vi "sub_main_mapgraph.vi"() -> (3 "graph ui array":T1(array[cluster]))   [LabVIEW 2019]
uses:
  Ctrl/waypoint_buf.ctl
  Ctrl/points.ctl
  Ctrl/pid-in-params.ctl
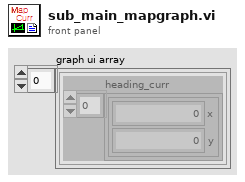
[diagram p1: front panel]
types:
  T1 = cluster{"heading_curr ":cluster{"x":dbl, "y":dbl}[]}[]
  T2 = cluster{"heading_curr ":cluster{"x":dbl, "y":dbl}[]}
  T3 = typedef "pid-in-params.ctl" = enum16{"read", "write"}
  T4 = typedef "points.ctl" = enum16{"read", "lookahead circle in", "lookahead in", "looktail in", "center in", "closest"}
  T5 = typedef "waypoint_buf.ctl" = enum16{"clear", "write", "read"}
  T6 = cluster{"deg_agv-lookahead":dbl, "deg_waypoint":dbl, "deg_gap":dbl, "deg_target":dbl, "pid output":dbl, "dis-gap":dbl, "deg_agv-center":dbl}
  T7 = cluster{"stop pt update out":cluster{dbl, dbl}[]}
  T8 = cluster{"waypoint out":cluster{"x":dbl, "y":dbl}[]}
  T9 = cluster{"lookahead circle out":cluster{"x":dbl, "y":dbl}[]}
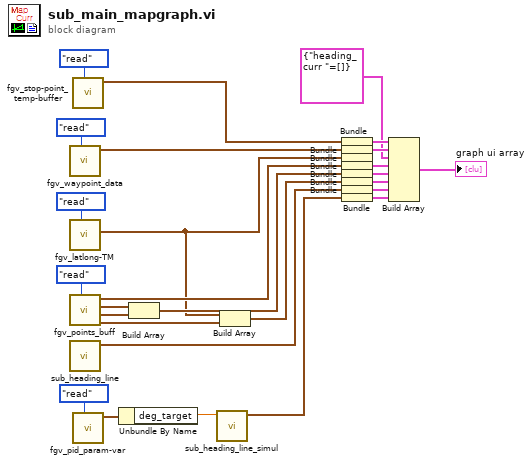
[diagram p0: block diagram]
diagram:
  n1 = call "fgv_waypoint_data.vi"("cmd"=waypoint_buf."read") -> ("waypoint out"=w8:cluster{"x":dbl, "y":dbl}[])  [unwired: 8 in, 2 out]
  n2 = call "fgv_latlong-TM.vi"("cmd"=enum16{"write", "read"}."read") -> ("latlong out"=w1:cluster{dbl, dbl})  [unwired: 9 in, 1 out]
  n3 = call "fgv_points_buff.vi"("cmd"=points."read") -> ("center out"=w9:cluster{"x":dbl, "y":dbl}, "looktail out"=w21:cluster{"x":dbl, "y":dbl}, "lookahead out"=w20:cluster{"x":dbl, "y":dbl}, "lookahead circle out"=w19:cluster{"x":dbl, "y":dbl}[])  [unwired: 6 in, 1 out]
  n4 = call "sub_heading_line.vi"() -> ("heading_curr"=w14:cluster{dbl, dbl}[])  [unwired: 11 in]
  n5 = call "fgv_stop-point_temp-buffer.vi"("cmd"=enum16{"init", "upload", "read", "del"}."read") -> ("stop pt update out"=w5:cluster{dbl, dbl}[])  [unwired: 10 in]
  n6 = call "fgv_pid_param-var.vi"("cmd"=pid-in-params."read") -> ("pid-var_output"=w4:T6)  [unwired: 10 in]
  n7 = Unbundle By Name(w4) -> ("deg_target"=w3:dbl)
  n8 = Build Array(w20, w21) -> (w23:cluster{"x":dbl, "y":dbl}[])
  n9 = call "sub_heading_line_simul.vi"("Heading"=w3) -> ("heading_curr"=w16:cluster{dbl, dbl}[])  [unwired: 9 in, 1 out]
  n10 = Build Array(w1, w9) -> (w24:cluster{"x":dbl, "y":dbl}[])
  n11 = Bundle("stop pt update out"=w5) -> (w7:T7)  [unwired: 1 in]
  n12 = Bundle("waypoint out"=w8) -> (w11:T8)  [unwired: 1 in]
  n13 = Bundle("latlong out"=w1) -> ()  [unwired: 1 in, 1 out]
  n14 = Bundle("lookahead circle out"=w19) -> (w13:T9)  [unwired: 1 in]
  n15 = Bundle(w23) -> (w22:cluster{cluster{"x":dbl, "y":dbl}[]})  [unwired: 1 in]
  n16 = Bundle(w24) -> (w25:cluster{cluster{"x":dbl, "y":dbl}[]})  [unwired: 1 in]
  n17 = Bundle("heading_curr"=w14) -> (w15:cluster{"heading_curr ":cluster{dbl, dbl}[]})  [unwired: 1 in]
  n18 = Bundle("heading_curr"=w16) -> (w17:cluster{"heading_curr ":cluster{dbl, dbl}[]})  [unwired: 1 in]
  n19 = Build Array(w7, w11, T2 {"heading_curr "=[]} ("element"), w13, w22, w25, w15, w17) -> (→"graph ui array":T1)
